vi "Configure Tracking.vi"(8 "error in (no error)":errorcluster, 10 "Track Channel (0: +25V Channel)":i32(ring) caption="Track Channel (0: +25V)" items=["+25V Channel", "-25V Channel", "Off"], 11 "VISA resource name":refnum<visa-resource-name>) -> (0 "error out":errorcluster, 3 "VISA resource name out":refnum<visa-resource-name>)   [LabVIEW 2020, in "RIGOL DP1000 Series.lvlib"]
doc: "Configures the channel track function."
uses:
  <instrlib>/RIGOL DP1000 Series/RIGOL DP1000 Series.lvlib
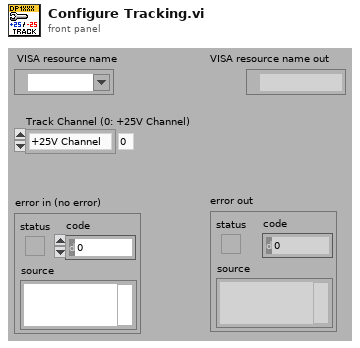
[diagram p1: front panel]
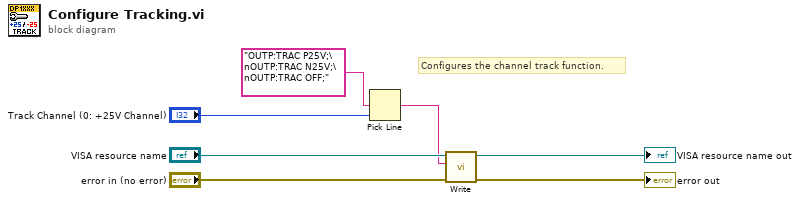
[diagram p0: block diagram]
diagram:
  # "Configures the channel track function."
  n1 = Pick Line(multi-line string="OUTP:TRAC P25V;\nOUTP:TRAC N25V;\nOUTP:TRAC OFF;", line index="Track Channel (0: +25V Channel)") -> (output string=w1:string)  [unwired: 1 out]
  n2 = call <instrlib>:"Write.vi"("error in (no error)"="error in (no error)", "Write Buffer (\"\")"=w1, "VISA resource name"="VISA resource name") -> ("error out"=→"error out":errorcluster, "VISA resource name out"=→"VISA resource name out":refnum<visa-resource-name>)  [unwired: 7 in]
